vi "Direction Correction.vi"(11 "Gyro Value":dbl) -> (3 "Z Value":dbl)   [LabVIEW 2014]
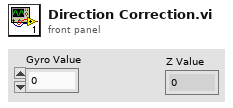
[diagram p1: front panel]
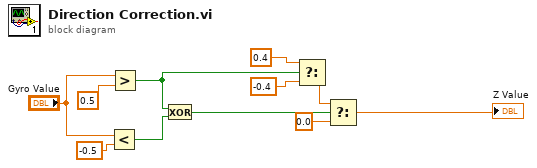
[diagram p0: block diagram]
diagram:
  n1 = Less?(x="Gyro Value", y=-0.5) -> (x < y?=w10:bool)
  n2 = Greater?(x="Gyro Value", y=0.5 ("x")) -> (0:w7:bool)
  n3 = Exclusive Or(1:w10, 2:w7) -> (0:w5:bool)
  n4 = Select(t=0.4, s=w7, f=-0.4) -> (s? t:f=w6:dbl)
  n5 = Select(t=w6, s=w5, f=0.0) -> (s? t:f=→"Z Value":dbl)
